vi "Add_Positions_to_stats.vi"(8 "Data row":string[](array[string]), 9 "No of stats columns":i32[](array[numeric]), 10 "Position":T1(array[cluster])=[{"Name"="LDA", "X"=999.9865969709155, "Y"=0.004861094232311693, "Z"=40.00084175084175}, {"Name"="CW", "X"=999.9865969709155, "Y"=0.004861094232311693, "Z"=40.00084175084175}, {"Name"="Gen", "X"=-2000.0, "Y"=200.0, "Z"=980.0}, {"Name"="T", "X"=999.9865969709155, "Y"=0.004861094232311693, "Z"=40.00084175084175}] {"Z" format="%.1f"; "Y" format="%.1f"; "X" format="%.1f"}) -> (0 "Data row with positions":string[](array[string]), 3 "row splitting":string[][](array[string]))   [LabVIEW 2010]
uses:
  Globals/Meas_global.vi
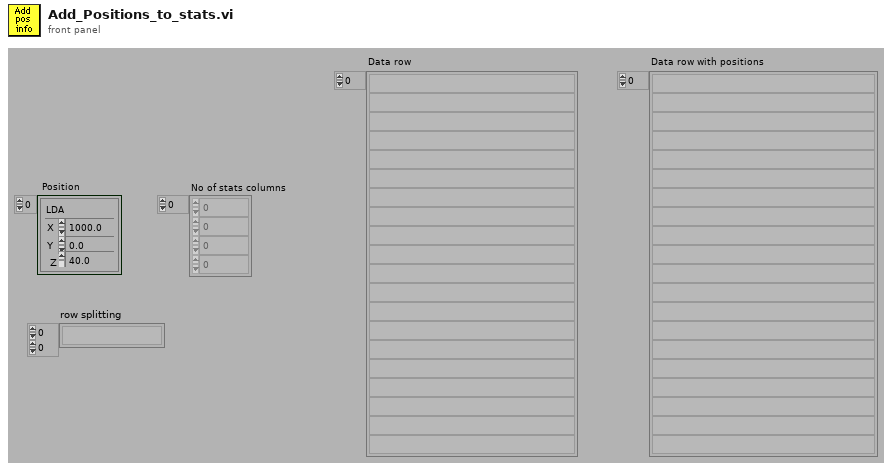
[diagram p1: front panel]
types:
  T1 = cluster{"Name":string, "X":dbl, "Y":dbl, "Z":dbl}[]
  T2 = cluster{"Name":string, "X":dbl, "Y":dbl, "Z":dbl}
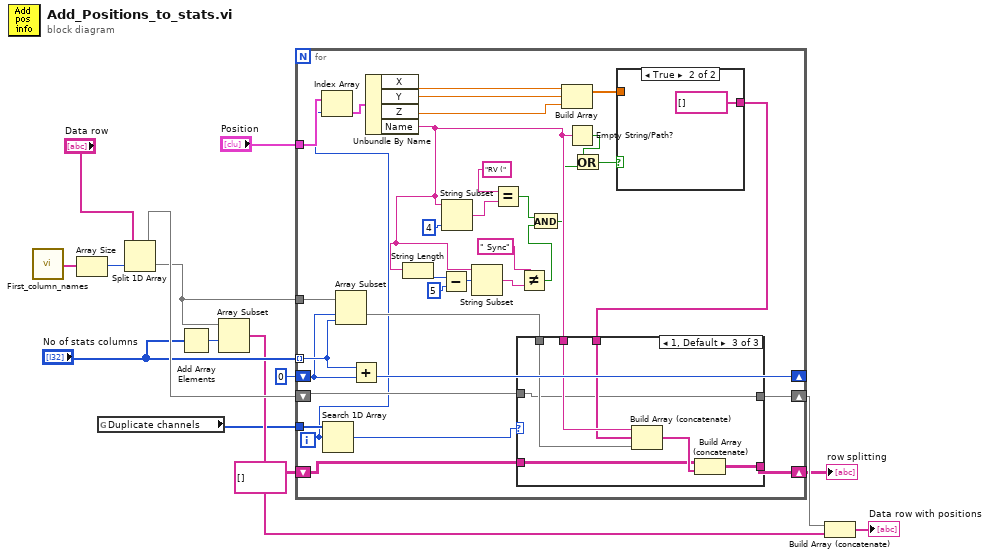
[diagram p0: block diagram]
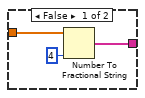
[diagram p2: hidden frame]
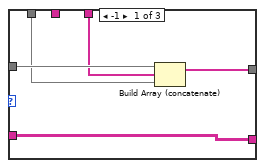
[diagram p3: hidden frame]
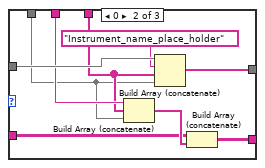
[diagram p4: hidden frame]
diagram:
  n1 = call "First_column_names.vi"() -> ("Array"=w4:string[])
  n2 = Array Size(array=w4) -> (size(s)=w12:i32)
  n3 = global read "Meas_global.vi" "Duplicate channels"() -> (w1:i32[])
  n4 = Split 1D Array(array="Data row", index=w12) -> (first subarray=w11:string[], second subarray=w6:string[])
  n5 = Add Array Elements(numeric array="No of stats columns") -> (sum=w7:i32)
  n6 = Array Subset(array=w6, index=w7) -> (w5:string[])  [unwired: 1 in]
  n7 = for {
    shift-right: [w46] -> w8
    shift-left: w11 -> [w47]
    tunnel: "Position" -> [w32]
    tunnel: "No of stats columns" -> [w45] mode=indexing
    tunnel: w6 -> [w48]
    shift-right: [w44] -> _
    shift-left: 0 -> [w43]
    tunnel: w1 -> [w36]
    shift-right: [w34] -> w2
    shift-left: string[][] [] -> [w33]
    i -> [w31]
    n8 = Index Array(array=w32, index=w31) -> (element=w30:T2)
    n9 = Search 1D Array(1D array=w36, element=w31) -> (index of element=w35:i32)  [unwired: 1 out]
    n10 = Array Subset(array=w48, index=w43, length=w45) -> (w38:string[])
    n11 = Add(x=w45, y=w43) -> (x+y=w44:i32)
    n12 = Unbundle By Name(w30) -> ("X"=w40:dbl, "Y"=w41:dbl, "Z"=w42:dbl, "Name"=w19:string)
    n13 = String Length(string=w19) -> (length=w24:i32)
    n14 = Subtract(x=w24, y=5) -> (x-y=w23:i32)
    n15 = String Subset(string=w19, length (rest)=4 ("length (rest)")) -> (substring=w28:string)  [unwired: 1 out]
    n16 = String Subset(string=w19, offset (0)=w23) -> (substring=w21:string)  [unwired: 1 out]
    n17 = Equal?(x="RV (", y=w28) -> (x = y?=w18:bool)
    n18 = Not Equal?(x=" Sync" ("substring"), y=w21) -> (x != y?=w17:bool)
    n19 = And(x=w18, y=w17) -> (x .and. y?=w16:bool)
    n20 = Build Array(w40, w41, w42) -> (w39:dbl[])
    n21 = Empty String/Path?(string/path=w19) -> (empty?=w26:bool)
    n22 = Or(x=w26, y=w16) -> (x .or. y?=w25:bool)
    n23 = case shown="True" w25 {
      tunnel: w39 -> [w50 _]
      tunnel: [w49 string[] []] -> w37
      frame False {
        n24 = Number To Fractional String(number=w50, precision (6)=i16 4) -> (F-format string=w49:string[])  [unwired: 2 out]
      }
      frame True {
      }
    }
    n25 = case shown="1, Default" w35 {
      tunnel: w47 -> [w57 w65 w67]
      tunnel: [w56 w66 w67] -> w46
      tunnel: w38 -> [w55 w61 w71]
      tunnel: w37 -> [w54 w62 w72]
      tunnel: w19 -> [_ w63 w73]
      tunnel: [w53 w59 w69] -> w34
      tunnel: w33 -> [w53 w58 w68]
      frame -1 {
        n26 = Build Array (concatenate)(w57, w54, w55) -> (w56:string[])
      }
      frame 0 {
        n27 = Build Array (concatenate)(w63, w62, w61) -> (w60:string[])
        n28 = Build Array (concatenate)(w65, "Instrument_name_place_holder", w62, w61) -> (w66:string[])
        n29 = Build Array (concatenate)(w58, w60) -> (w59:string[][])
      }
      frame 1, Default {
        n30 = Build Array (concatenate)(w73, w72, w71) -> (w70:string[])
        n31 = Build Array (concatenate)(w68, w70) -> (w69:string[][])
      }
    }
  }
  "row splitting" <- w2
  n32 = Build Array (concatenate)(w8, w5) -> (→"Data row with positions":string[])
